vi "Request.vi"(6 "Response":bool, 8 "error in (no error)":errorcluster, 9 "Data":string, 10 "Function ID":u8, 11 "Device in":refnum<class "Device.lvclass">) -> (0 "error out":errorcluster, 1 "Sucessful":bool, 2 "Answer":T1, 3 "Device out":refnum<class "Device.lvclass">, 4 "timed out":bool)   [LabVIEW 2011, in "Tinkerforge.lvlib" / "Device.lvclass"]
doc: "This VI encapsulates the request SubVI of the IP connection class for all child class implementations."
uses:
  Device.lvclass
  IP Connection/Type Definitions/Answer.ctl
  IP Connection/Type Definitions/Request Type.ctl
  Device.lvclass/Device.ctl
  IP Connection/IP Connection.lvclass
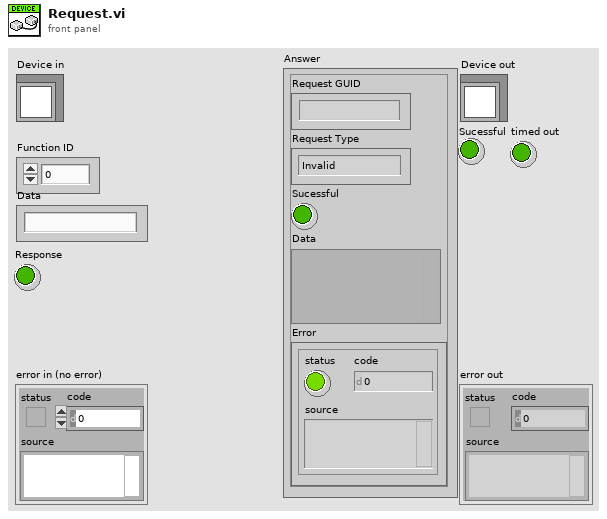
[diagram p1: front panel]
types:
  T1 = typedef "Tinkerforge.lvlib/IP Connection.lvclass/Answer.ctl" = cluster{"Request GUID":string, "Request Type":T2, "Sucessful":bool, "Data":variant, "Error":errorcluster}
  T2 = typedef "Tinkerforge.lvlib/IP Connection.lvclass/Request Type.ctl" = enum8{"Invalid", "Write"}
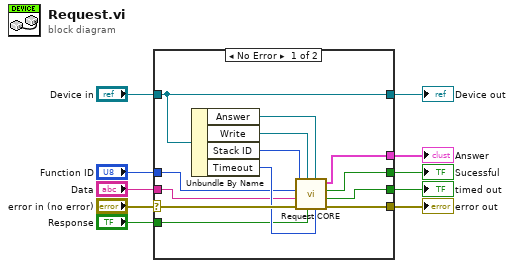
[diagram p0: block diagram]
diagram:
  n1 = case shown="No Error" "error in (no error)" {
    selector: "error in (no error)" -> [w23 w25]
    tunnel: [w22 w25] -> w9
    tunnel: [w21 w24] -> w7
    tunnel: "Device in" -> [w21 w24]
    tunnel: "Function ID" -> [w16 _]
    tunnel: "Data" -> [w15 _]
    tunnel: "Response" -> [w14 _]
    tunnel: [w11 _] -> w3
    tunnel: [w12 _] -> w2
    tunnel: [w13 _] -> w1
    frame No Error {
      n2 = Unbundle By Name(w21) -> ("Answer"=w20:refnum<user-event>, "Write"=w19:refnum<queue>, "Stack ID"=w18:u8, "Timeout"=w17:i32)
      n3 = call "Request CORE.vi"("Timeout"=w17, "Answer UE"=w20, "Response"=w14, "Write"=w19, "Error In"=w23, "Data"=w15, "Function ID"=w16, "Stack ID"=w18) -> ("Error Out"=w22:errorcluster, "timed out"=w11:bool, "Sucessful"=w12:bool, "Answer"=w13:T1)
    }
    frame Error {
    }
  }
  "error out" <- w9
  "Device out" <- w7
  "Answer" <- w1
  "Sucessful" <- w2
  "timed out" <- w3
